vi "Generate Trace.vi"(10 "Trace String":string, 11 "DETT Format in":refnum<class "DETT Format.lvclass">) -> (3 "DETT Format out":refnum<class "DETT Format.lvclass">)   [LabVIEW 2020, in "AF Debug.lvlib" / "DETT Format.lvclass"]
uses:
  DETT Format.lvclass
  DETT Format.lvclass/DETT Format.ctl
  <vilib>/Utility/SystemLogging/NI_SystemLogging.lvlib
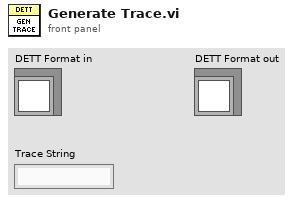
[diagram p1: front panel]
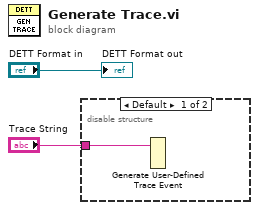
[diagram p0: block diagram]
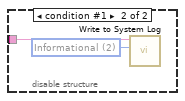
[diagram p2: hidden frame]
diagram:
  n1 = disable-structure shown="Default" {
    disable-tunnel: "Trace String" -> [w3 w5]
    frame condition #0 (active) {
      n2 = Generate User-Defined Trace Event(2:w3) -> ()  [unwired: 1 in]
    }
    frame condition #1 {
      w4 = 2 items=["Error", "Warning", "Informational"] ("severity")
      n3 = call <vilib>:"Write to System Log.vi"("severity"=w4, "message"=w5) -> ()  [unwired: 9 in, 1 out]
    }
  }
  "DETT Format out" <- "DETT Format in"
